vi "Untitled 2.vi"() -> ()   [LabVIEW 2020]
panel:
  out "agotado 3":string="Articulo agotado"
  in  "# dulce":dbl
  in  "#bebida fria":dbl
  in  "#cafe":dbl
  in  "# snack":dbl
  in  "stop":bool
  in  "Tab Control":enum32{"Page 1", "Page 2"}(tab)
  out "producto":bool
  out "cambio":bool
  in  "dulce":bool
  in  "bebida fria":bool
  in  "cafe":bool
  in  "snack":bool
  in  "Cancelar":bool
  in  "comprar":bool
  in  "Monedas":cluster{"moneda 10":bool, "moneda 20":bool}
  out "Cambio":dbl
  out "Dinero ingresado":dbl
  out "agotado":string="Articulo agotado"
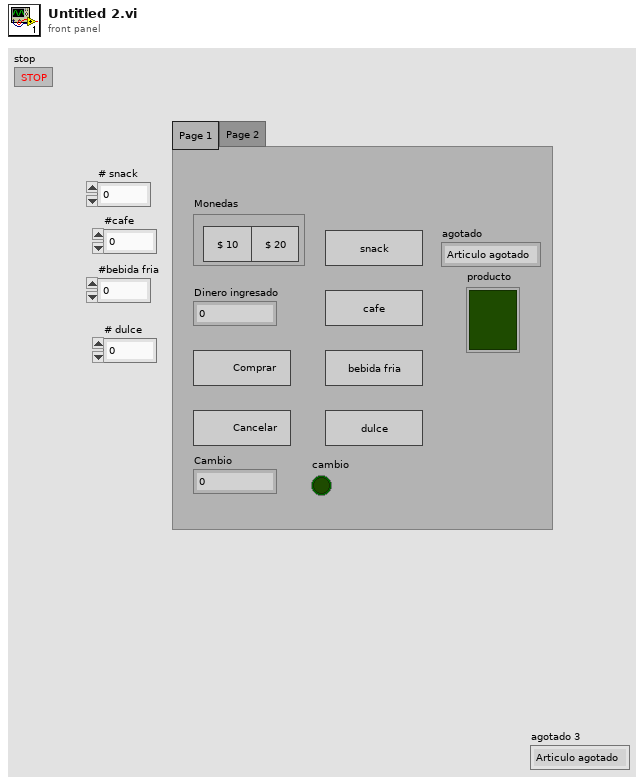
[diagram p1: front panel]
types:
  T1 = enum16{"inicio", "snack", "comprar s", "cambio s", "cafe", "comprar c", "cambio c", "bebida fria", "comprar bf", "cambio bf", "dulce", "comprar d", "cambio d", "reinicio", "cancelar"}
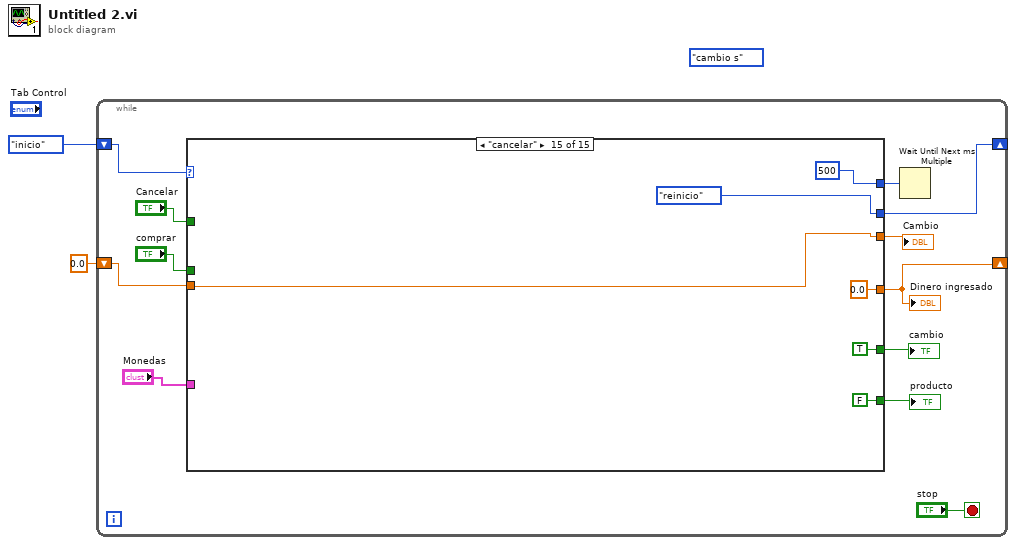
[diagram p0: block diagram]
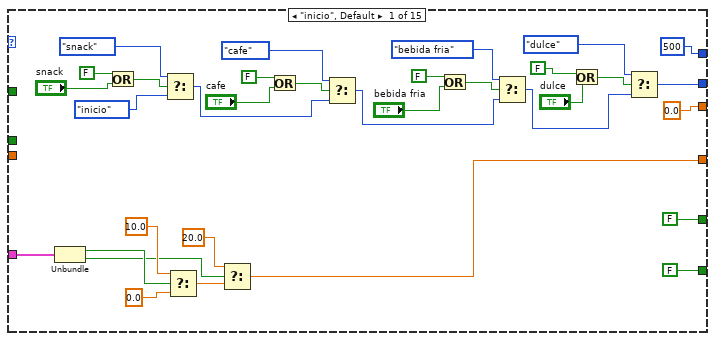
[diagram p2: hidden frame]
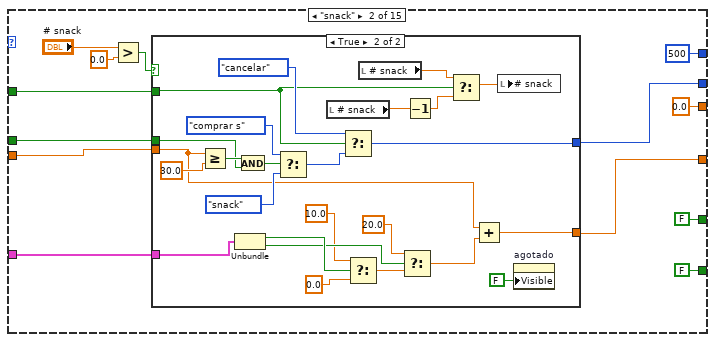
[diagram p3: hidden frame]
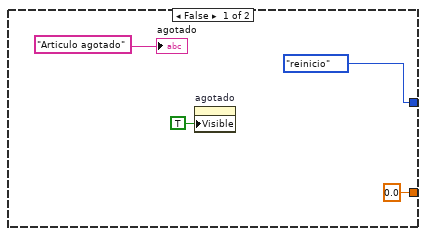
[diagram p4: hidden frame]
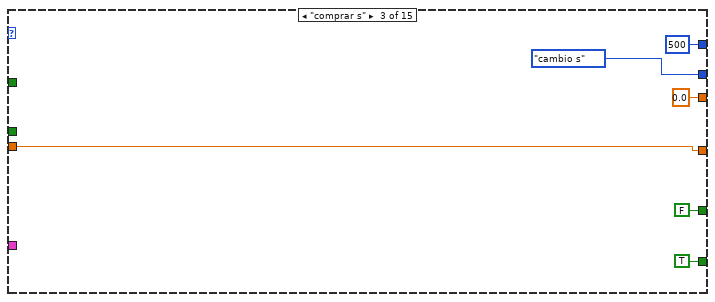
[diagram p5: hidden frame]
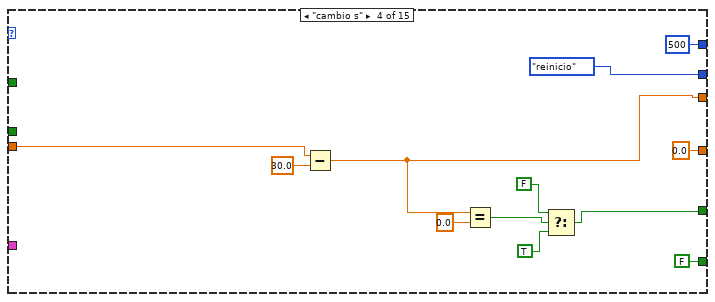
[diagram p6: hidden frame]
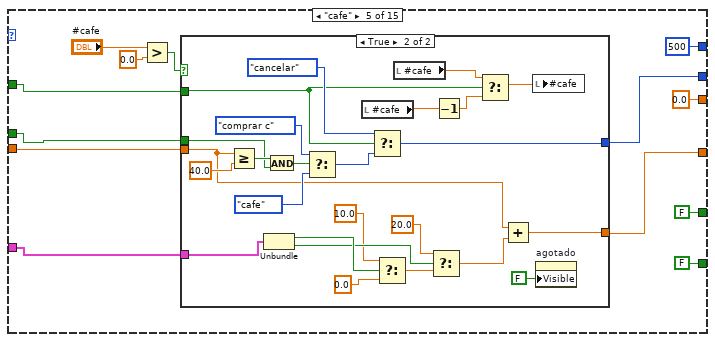
[diagram p7: hidden frame]
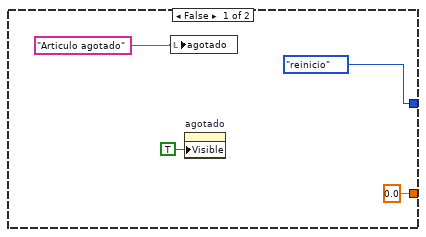
[diagram p8: hidden frame]
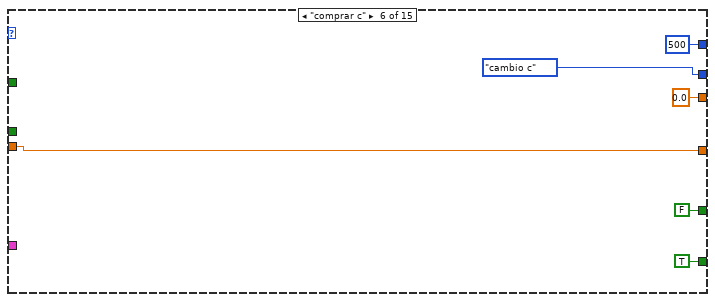
[diagram p9: hidden frame]
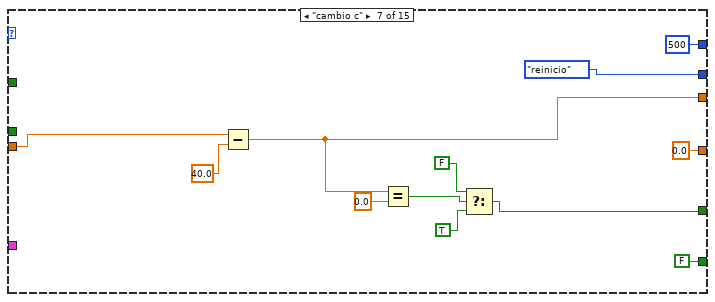
[diagram p10: hidden frame]
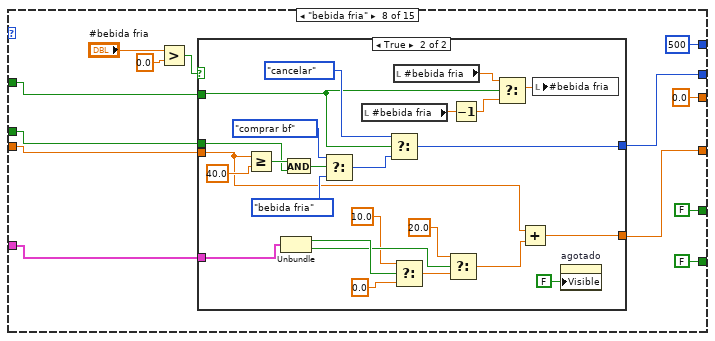
[diagram p11: hidden frame]
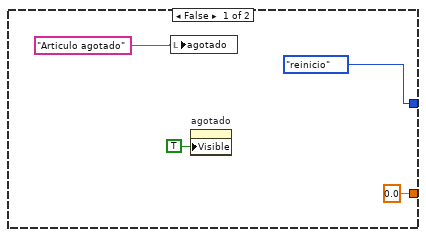
[diagram p12: hidden frame]
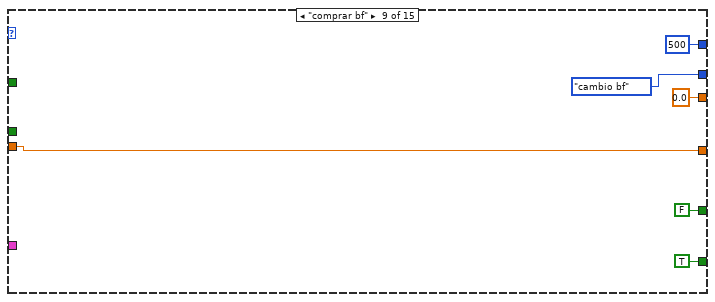
[diagram p13: hidden frame]
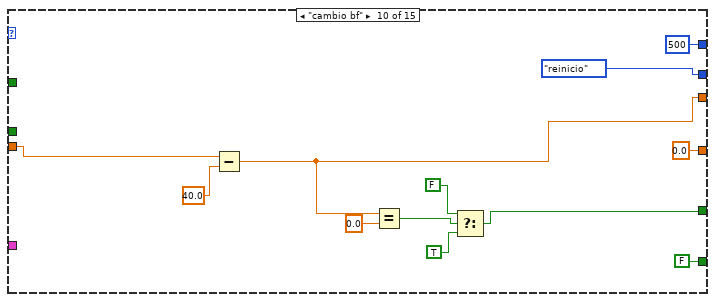
[diagram p14: hidden frame]
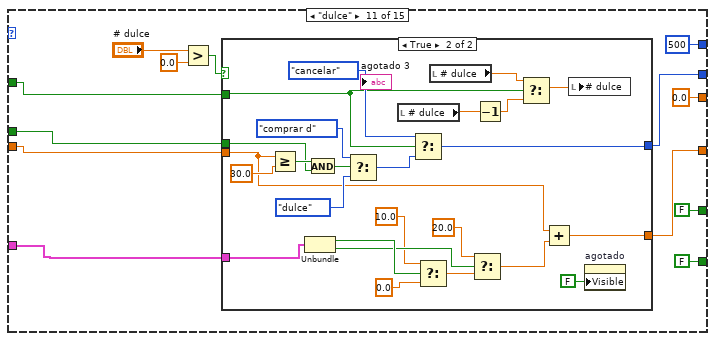
[diagram p15: hidden frame]
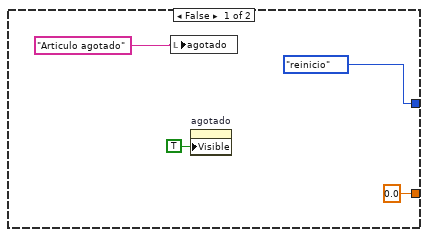
[diagram p16: hidden frame]
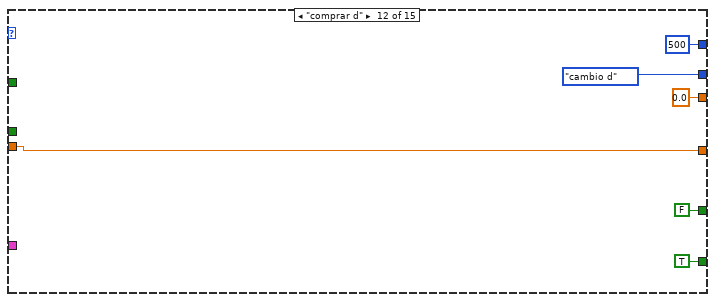
[diagram p17: hidden frame]
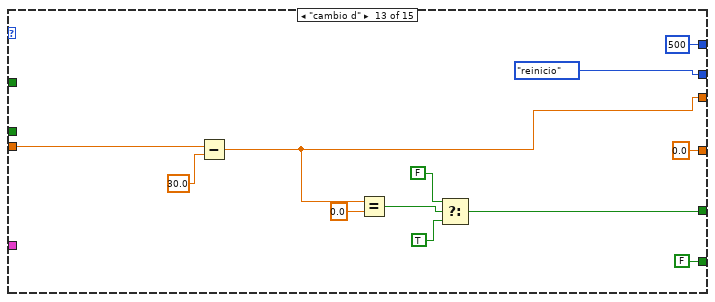
[diagram p18: hidden frame]
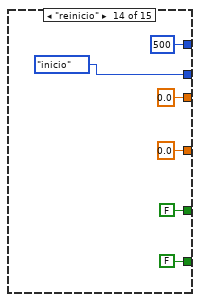
[diagram p19: hidden frame]
diagram:
  (unwired) T1."cambio s"
  n1 = while {
    shift-right: [w12] -> _
    shift-left: T1."inicio" -> [w14]
    shift-right: [w6] -> _
    shift-left: 0.0 ("f") -> [w5]
    stop <- "stop" stop-if-true
    n2 = case shown="\"cancelar\"" w14 {
      tunnel: [500 500 500 500 500 500 500 500 500 500 500 500 500 500 500] -> w13
      tunnel: [w26 w52 T1."cambio s" T1."reinicio" w113 T1."cambio c" T1."reinicio" w173 T1."cambio bf" T1."reinicio" w232 T1."cambio d" T1."reinicio" T1."inicio" T1."reinicio"] -> w12
      tunnel: [0.0 0.0 0.0 w104 0.0 0.0 w158 0.0 0.0 w220 0.0 0.0 w279 0.0 w297] -> w11
      tunnel: "Monedas" -> [w24 w54 _ _ w114 _ _ w174 _ _ w237 _ _ _ _]
      tunnel: [w17 w53 w92 0.0 ("f") w112 w155 0.0 ("f") w170 w212 0.0 ("f") w231 w272 0.0 ("f") 0.0 ("f") 0.0 ("f")] -> w6
      tunnel: [FALSE FALSE TRUE FALSE FALSE TRUE FALSE FALSE TRUE FALSE FALSE TRUE FALSE FALSE FALSE] -> w9
      tunnel: [FALSE FALSE FALSE w100 FALSE FALSE w160 FALSE FALSE w218 FALSE FALSE w278 FALSE TRUE] -> w8
      tunnel: w5 -> [_ w57 w92 w107 w115 w155 w156 w175 w212 w216 w236 w272 w276 _ w297]
      tunnel: "comprar" -> [_ w56 _ _ w116 _ _ w176 _ _ w235 _ _ _ _]
      tunnel: "Cancelar" -> [_ w55 _ _ w117 _ _ w177 _ _ w234 _ _ _ _]
      frame "inicio", Default {
        n3 = Unbundle(w24) -> ("moneda 10"=w23:bool, "moneda 20"=w19:bool)
        n4 = Or(x=FALSE, y="snack") -> (x .or. y?=w45:bool)
        n5 = Select(t=T1."snack", s=w45, f=T1."inicio") -> (s? t:f=w38:T1)
        n6 = Select(t=10.0, s=w23, f=0.0) -> (s? t:f=w20:dbl)
        n7 = Select(t=20.0, s=w19, f=w20) -> (s? t:f=w17:dbl)
        n8 = Or(x=FALSE, y="cafe") -> (x .or. y?=w41:bool)
        n9 = Select(t=T1."cafe", s=w41, f=w38) -> (s? t:f=w33:T1)
        n10 = Or(x=FALSE, y="bebida fria") -> (x .or. y?=w36:bool)
        n11 = Select(t=T1."bebida fria", s=w36, f=w33) -> (s? t:f=w28:T1)
        n12 = Or(x=FALSE, y="dulce") -> (x .or. y?=w31:bool)
        n13 = Select(t=T1."dulce", s=w31, f=w28) -> (s? t:f=w26:T1)
      }
      frame "snack" {
        n14 = Greater?(x="# snack", y=0.0) -> (0:w58:bool)
        n15 = case shown="True" w58 {
          tunnel: w57 -> [_ w73]
          tunnel: w56 -> [_ w84]
          tunnel: w55 -> [_ w71]
          tunnel: w54 -> [_ w75]
          tunnel: [0.0 w72] -> w53
          tunnel: [T1."reinicio" w66] -> w52
          frame False {
            n16 = property on="agotado" class="Str"("Visible"=TRUE) -> ()  [unwired: 2 in, 2 out]
            "agotado" <- "Articulo agotado"
          }
          frame True {
            n17 = Greater Or Equal?(x=w73, y=30.0) -> (x >= y?=w88:bool)
            n18 = Unbundle(w75) -> ("moneda 10"=w81:bool, "moneda 20"=w79:bool)
            n19 = And(x=w88, y=w84) -> (x .and. y?=w89:bool)
            n20 = Select(t=T1."comprar s", s=w89, f=T1."snack") -> (s? t:f=w83:T1)
            n21 = local read "# snack"() -> (w70:dbl)
            n22 = Select(t=T1."cancelar", s=w71, f=w83) -> (s? t:f=w66:T1)
            n23 = Select(t=10.0, s=w81, f=0.0) -> (s? t:f=w80:dbl)
            n24 = local read "# snack"() -> (w67:dbl)
            n25 = Select(t=20.0, s=w79, f=w80) -> (s? t:f=w74:dbl)
            n26 = Decrement(x=w70) -> (x-1=w69:dbl)
            n27 = Select(t=w67, s=w71, f=w69) -> (s? t:f=w68:dbl)
            n28 = Add(x=w73, y=w74) -> (x+y=w72:dbl)
            n29 = local write "# snack"(w68) -> ()
            n30 = property on="agotado" class="Str"("Visible"=FALSE) -> ()  [unwired: 2 in, 2 out]
          }
        }
      }
      frame "comprar s" {
      }
      frame "cambio s" {
        n31 = Subtract(x=w107, y=30.0) -> (x-y=w104:dbl)
        n32 = Equal?(x=w104, y=0.0) -> (x = y?=w102:bool)
        n33 = Select(t=FALSE, s=w102, f=TRUE) -> (s? t:f=w100:bool)
      }
      frame "cafe" {
        n34 = Greater?(x="#cafe", y=0.0) -> (0:w118:bool)
        n35 = case shown="True" w118 {
          tunnel: w115 -> [_ w133]
          tunnel: w116 -> [_ w144]
          tunnel: w117 -> [_ w131]
          tunnel: w114 -> [_ w135]
          tunnel: [0.0 w132] -> w112
          tunnel: [T1."reinicio" w126] -> w113
          frame False {
            n36 = local write "agotado"("Articulo agotado") -> ()
            n37 = property on="agotado" class="Str"("Visible"=TRUE) -> ()  [unwired: 2 in, 2 out]
          }
          frame True {
            n38 = Greater Or Equal?(x=w133, y=40.0) -> (x >= y?=w148:bool)
            n39 = Unbundle(w135) -> ("moneda 10"=w141:bool, "moneda 20"=w139:bool)
            n40 = And(x=w148, y=w144) -> (x .and. y?=w149:bool)
            n41 = Select(t=T1."comprar c", s=w149, f=T1."cafe") -> (s? t:f=w143:T1)
            n42 = local read "#cafe"() -> (w130:dbl)
            n43 = Select(t=T1."cancelar", s=w131, f=w143) -> (s? t:f=w126:T1)
            n44 = Select(t=10.0, s=w141, f=0.0) -> (s? t:f=w140:dbl)
            n45 = local read "#cafe"() -> (w127:dbl)
            n46 = Select(t=20.0, s=w139, f=w140) -> (s? t:f=w134:dbl)
            n47 = Decrement(x=w130) -> (x-1=w129:dbl)
            n48 = Select(t=w127, s=w131, f=w129) -> (s? t:f=w128:dbl)
            n49 = Add(x=w133, y=w134) -> (x+y=w132:dbl)
            n50 = local write "#cafe"(w128) -> ()
            n51 = property on="agotado" class="Str"("Visible"=FALSE) -> ()  [unwired: 2 in, 2 out]
          }
        }
      }
      frame "comprar c" {
      }
      frame "cambio c" {
        n52 = Subtract(x=w156, y=40.0) -> (x-y=w158:dbl)
        n53 = Equal?(x=w158, y=0.0) -> (x = y?=w163:bool)
        n54 = Select(t=FALSE, s=w163, f=TRUE) -> (s? t:f=w160:bool)
      }
      frame "bebida fria" {
        n55 = Greater?(x="#bebida fria", y=0.0) -> (0:w178:bool)
        n56 = case shown="True" w178 {
          tunnel: w175 -> [_ w193]
          tunnel: w176 -> [_ w204]
          tunnel: w177 -> [_ w191]
          tunnel: w174 -> [_ w195]
          tunnel: [0.0 w192] -> w170
          tunnel: [T1."reinicio" w186] -> w173
          frame False {
            n57 = local write "agotado"("Articulo agotado") -> ()
            n58 = property on="agotado" class="Str"("Visible"=TRUE) -> ()  [unwired: 2 in, 2 out]
          }
          frame True {
            n59 = Greater Or Equal?(x=w193, y=40.0) -> (x >= y?=w208:bool)
            n60 = Unbundle(w195) -> ("moneda 10"=w201:bool, "moneda 20"=w199:bool)
            n61 = And(x=w208, y=w204) -> (x .and. y?=w209:bool)
            n62 = Select(t=T1."comprar bf", s=w209, f=T1."bebida fria") -> (s? t:f=w203:T1)
            n63 = local read "#bebida fria"() -> (w190:dbl)
            n64 = Select(t=T1."cancelar", s=w191, f=w203) -> (s? t:f=w186:T1)
            n65 = local read "#bebida fria"() -> (w187:dbl)
            n66 = Select(t=10.0, s=w201, f=0.0) -> (s? t:f=w200:dbl)
            n67 = Select(t=20.0, s=w199, f=w200) -> (s? t:f=w194:dbl)
            n68 = Decrement(x=w190) -> (x-1=w189:dbl)
            n69 = Select(t=w187, s=w191, f=w189) -> (s? t:f=w188:dbl)
            n70 = Add(x=w193, y=w194) -> (x+y=w192:dbl)
            n71 = local write "#bebida fria"(w188) -> ()
            n72 = property on="agotado" class="Str"("Visible"=FALSE) -> ()  [unwired: 2 in, 2 out]
          }
        }
      }
      frame "comprar bf" {
      }
      frame "cambio bf" {
        n73 = Subtract(x=w216, y=40.0) -> (x-y=w220:dbl)
        n74 = Equal?(x=w220, y=0.0) -> (x = y?=w223:bool)
        n75 = Select(t=FALSE, s=w223, f=TRUE) -> (s? t:f=w218:bool)
      }
      frame "dulce" {
        n76 = Greater?(x="# dulce", y=0.0) -> (0:w239:bool)
        n77 = case shown="True" w239 {
          tunnel: w236 -> [_ w253]
          tunnel: w235 -> [_ w264]
          tunnel: w234 -> [_ w251]
          tunnel: w237 -> [_ w255]
          tunnel: [0.0 w252] -> w231
          tunnel: [T1."reinicio" w246] -> w232
          frame False {
            n78 = local write "agotado"("Articulo agotado") -> ()
            n79 = property on="agotado" class="Str"("Visible"=TRUE) -> ()  [unwired: 2 in, 2 out]
          }
          frame True {
            n80 = Greater Or Equal?(x=w253, y=30.0) -> (x >= y?=w268:bool)
            n81 = Unbundle(w255) -> ("moneda 10"=w261:bool, "moneda 20"=w259:bool)
            n82 = And(x=w268, y=w264) -> (x .and. y?=w269:bool)
            n83 = Select(t=T1."comprar d", s=w269, f=T1."dulce") -> (s? t:f=w263:T1)
            n84 = local read "# dulce"() -> (w250:dbl)
            n85 = Select(t=T1."cancelar", s=w251, f=w263) -> (s? t:f=w246:T1)
            n86 = Select(t=10.0, s=w261, f=0.0) -> (s? t:f=w260:dbl)
            n87 = local read "# dulce"() -> (w247:dbl)
            n88 = Select(t=20.0, s=w259, f=w260) -> (s? t:f=w254:dbl)
            n89 = Decrement(x=w250) -> (x-1=w249:dbl)
            n90 = Select(t=w247, s=w251, f=w249) -> (s? t:f=w248:dbl)
            n91 = Add(x=w253, y=w254) -> (x+y=w252:dbl)
            n92 = local write "# dulce"(w248) -> ()
            n93 = property on="agotado" class="Str"("Visible"=FALSE) -> ()  [unwired: 2 in, 2 out]
          }
        }
      }
      frame "comprar d" {
      }
      frame "cambio d" {
        n94 = Subtract(x=w276, y=30.0) -> (x-y=w279:dbl)
        n95 = Equal?(x=w279, y=0.0) -> (x = y?=w282:bool)
        n96 = Select(t=FALSE, s=w282, f=TRUE) -> (s? t:f=w278:bool)
      }
      frame "reinicio" {
      }
      frame "cancelar" {
      }
    }
    "Cambio" <- w11
    "Dinero ingresado" <- w6
    "cambio" <- w8
    "producto" <- w9
    n97 = Wait Until Next ms Multiple(millisecond multiple=w13) -> ()  [unwired: 1 out]
  }
